vi "Thermostat.vi"() -> ()   [LabVIEW 2025]
panel:
  out "Week day":string
  out "Time":string
  out "Date":string
  out "Desired Temp":dbl format="%#_3g"
  out "Heater on":bool
  out "Room name":string
  out "Current Temp":dbl format="%#_3g"
  in  "STOP":bool
  in  "DOWN":bool
  in  "UP":bool
  in  "Room select":i32 min=0 max=3
  # "Set"
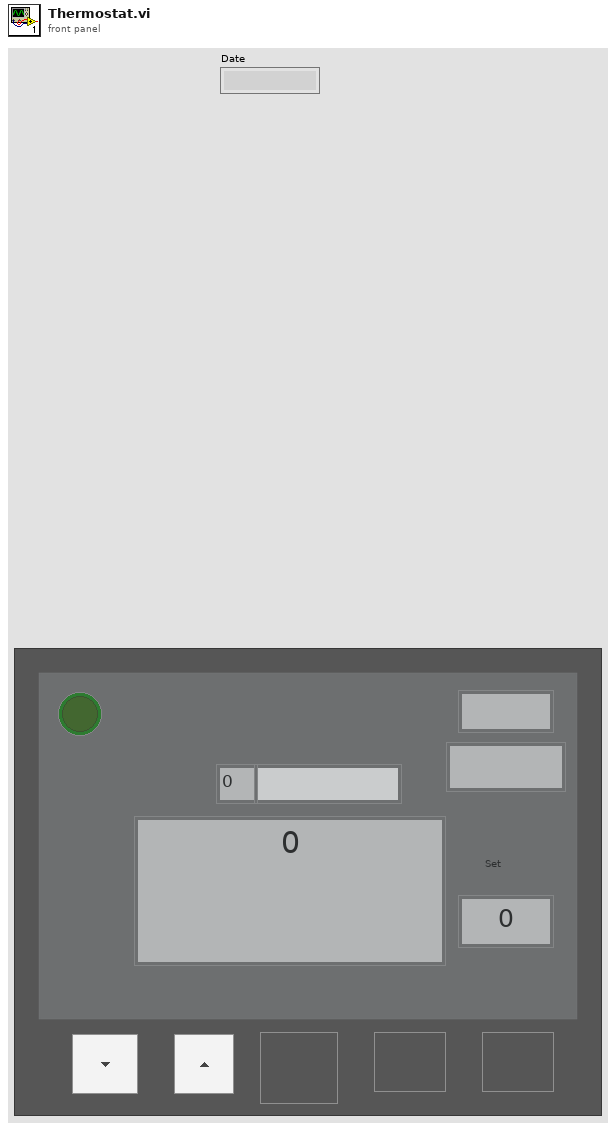
[diagram p1: front panel]
types:
  T1 = cluster{"Room name":string, "Desired Temp":dbl, "Current Temp":dbl, "Heater on":bool}[]
  T2 = cluster{"Room name":string, "Desired Temp":dbl, "Current Temp":dbl, "Heater on":bool}
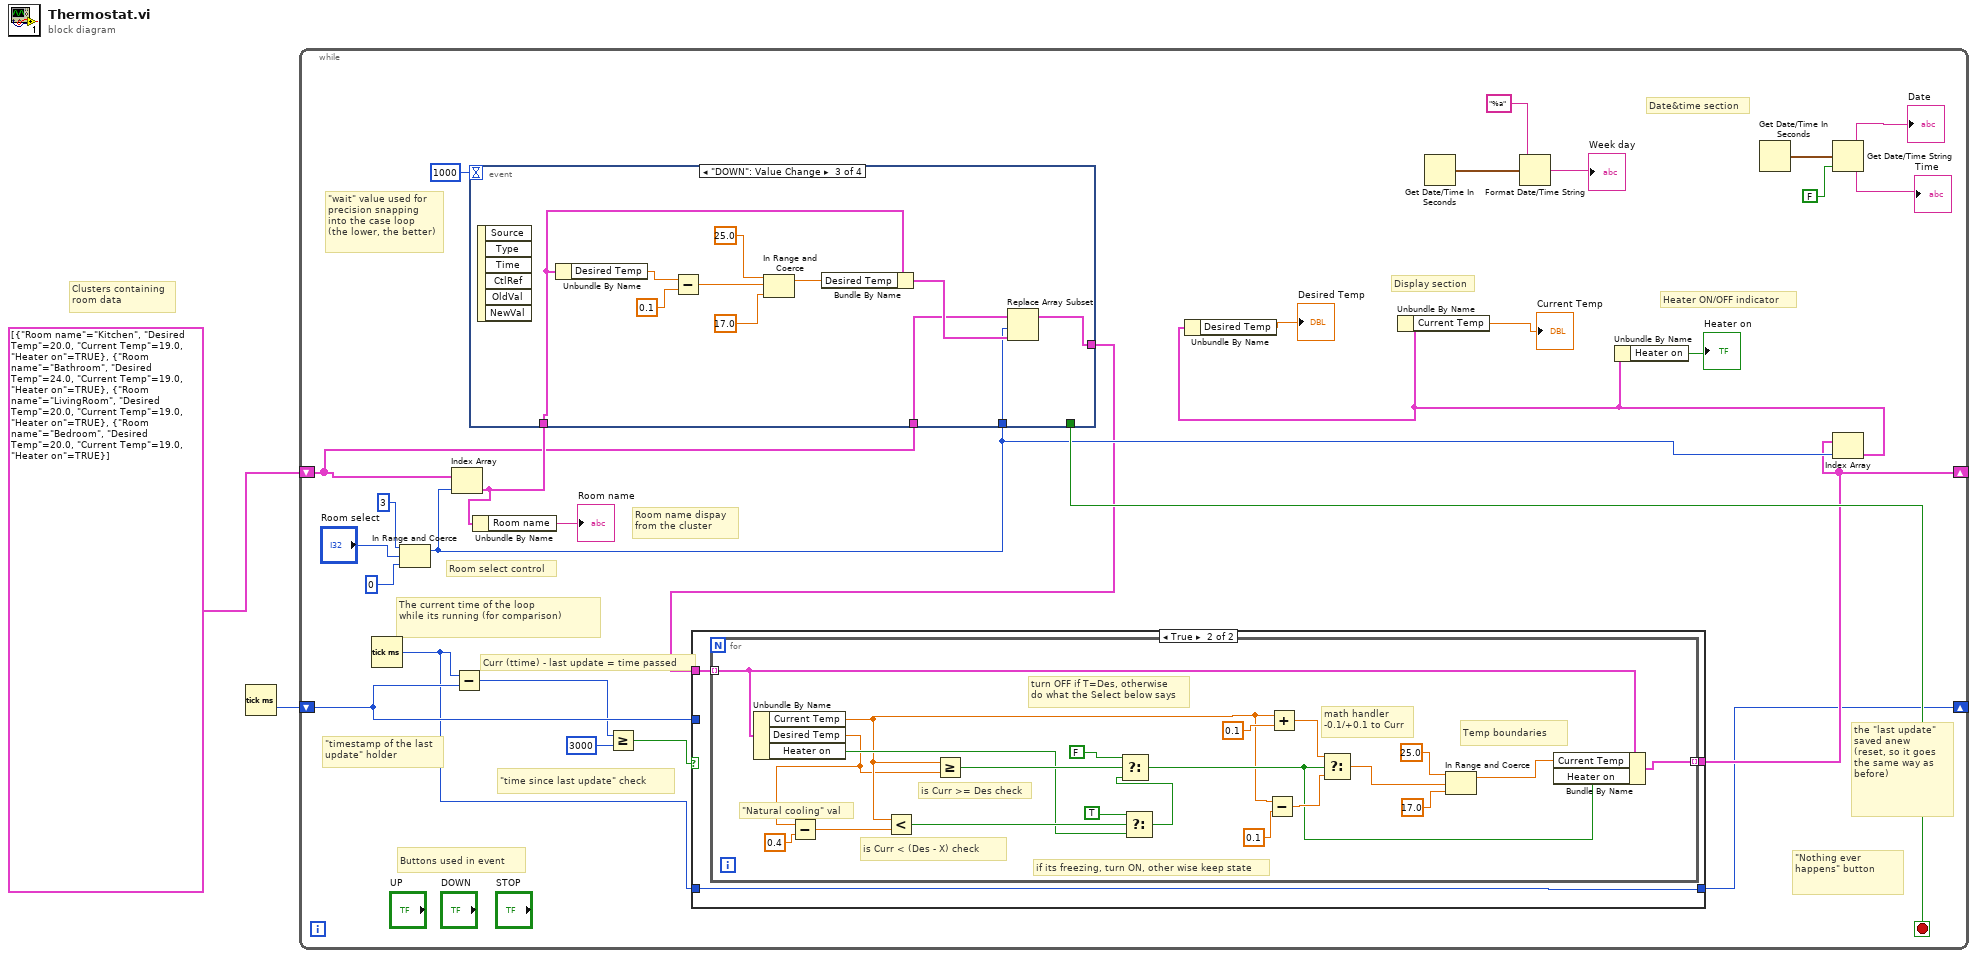
[diagram p0: block diagram]
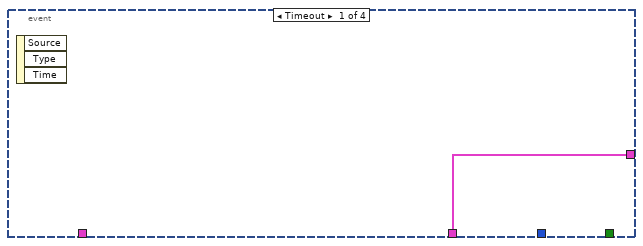
[diagram p3: hidden frame]
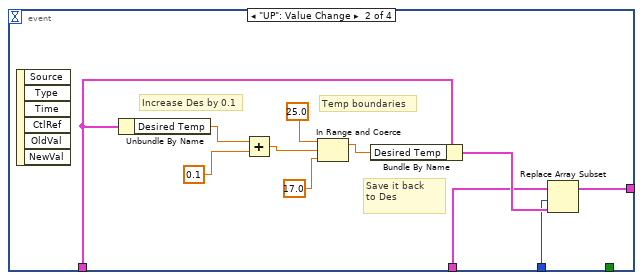
[diagram p4: hidden frame]
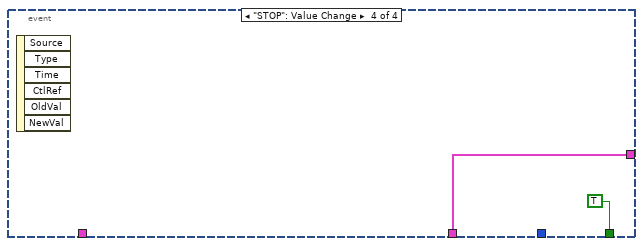
[diagram p5: hidden frame]
diagram:
  # "Clusters containing\nroom data"
  n1 = Tick Count (ms)() -> (millisecond timer value=w1:u32)
  n2 = while {
    shift-right: [w19] -> _
    shift-left: T1 [{"Room name"="Kitchen", "Desired Temp"=20.0, "Current Temp"=19.0, "Heater on"=TRUE}, {"Room name"="Bathroom", "Desired Temp"=24.0, "Current Temp"=19.0, "Heater on"=TRUE}, {"Room name"="LivingRoom", "Desired Temp"=20.0, "Current Temp"=19.0, "Heater on"=TRUE}, {"Room name"="Bedroom", "Desired Temp"=20.0, "Current Temp"=19.0, "Heater on"=TRUE}] -> [w20]
    shift-right: [w14] -> _
    shift-left: w1 -> [w16]
    stop <- w28 stop-if-true
    # "Heater ON/OFF indicator"
    # "Date&time section"
    # "Room select control"
    # "\"timestamp of the last\nupdate\" holder"
    # "\"wait\" value used for\nprecision snapping\ninto the case loop\n(the lower, the better)"
    # "the \"last update\"\nsaved anew\n(reset, so it goes\nthe same way as\nbefore)"
    # "\"time since last update\" check"
    # "Curr (ttime) - last update = time passed"
    # "The current time of the loop\nwhile its running (for comparison)"
    # "Buttons used in event"
    # "Room name dispay\nfrom the cluster"
    # "\"Nothing ever\nhappens\" button"
    # "Display section"
    n3 = Tick Count (ms)() -> (millisecond timer value=w13:u32)
    n4 = In Range and Coerce(upper limit=3, x="Room select", lower limit=0) -> (coerced(x)=w22:i32)  [unwired: 1 out]
    n5 = Index Array(array=w20, index=w22) -> (element=w23:T2)
    n6 = Subtract(x=w13, y=w16) -> (x-y=w15:u32)
    n7 = event shown="[2] \"DOWN\": Value Change" {
      selector: _ -> [_ _ _ _]
      dyn-events: _ -> [_ _ _ _]
      timeout: 1000 -> [_ _ _ _]
      tunnel: w23 -> [_ w63 w74 _]
      tunnel: [w57 w58 w70 w80] -> w12
      tunnel: w22 -> [_ w59 w69 _]
      tunnel: w20 -> [w57 w60 w71 w80]
      tunnel: [_ _ _ TRUE] -> w28
      event Timeout {
        n8 = event-data() -> ()  [unwired: 1 in, 3 out]
      }
      event "UP": Value Change {
        # "Save it back\nto Des"
        # "Increase Des by 0.1"
        # "Temp boundaries"
        n9 = event-data() -> ()  [unwired: 1 in, 6 out]
        n10 = Unbundle By Name(w63) -> ("Desired Temp"=w67:dbl)
        n11 = Add(x=w67, y=0.1) -> (x+y=w66:dbl)
        n12 = In Range and Coerce(upper limit=25.0, x=w66, lower limit=17.0) -> (coerced(x)=w62:dbl)  [unwired: 1 out]
        n13 = Bundle By Name(cluster=w63, "Desired Temp"=w62) -> (w61:T2)
        n14 = Replace Array Subset(array=w60, new element=w61, index=w59) -> (w58:T1)
      }
      event "DOWN": Value Change {
        n15 = event-data() -> ()  [unwired: 1 in, 6 out]
        n16 = Unbundle By Name(w74) -> ("Desired Temp"=w78:dbl)
        n17 = Subtract(x=w78, y=0.1) -> (x-y=w77:dbl)
        n18 = In Range and Coerce(upper limit=25.0, x=w77, lower limit=17.0) -> (coerced(x)=w73:dbl)  [unwired: 1 out]
        n19 = Bundle By Name(cluster=w74, "Desired Temp"=w73) -> (w72:T2)
        n20 = Replace Array Subset(array=w71, new element=w72, index=w69) -> (w70:T1)
      }
      event "STOP": Value Change {
        n21 = event-data() -> ()  [unwired: 1 in, 6 out]
      }
    }
    n22 = Unbundle By Name(w23) -> ("Room name"=→"Room name":string)
    n23 = Greater Or Equal?(x=w15, y=u32 3000) -> (x >= y?=w17:bool)
    n24 = case shown="True" w17 {
      tunnel: w12 -> [w32 w35]
      tunnel: [w32 w34] -> w19
      tunnel: w16 -> [w31 _]
      tunnel: w13 -> [_ w33]
      tunnel: [w31 w33] -> w14
      frame False {
      }
      frame True {
        n25 = for {
          tunnel: w35 -> [w39] mode=indexing
          tunnel: [w53] -> w34 mode=indexing
          # "Temp boundaries"
          # "math handler\n-0.1/+0.1 to Curr"
          # "turn OFF if T=Des, otherwise\ndo what the Select below says"
          # "if its freezing, turn ON, other wise keep state"
          # "\"Natural cooling\" val"
          # "is Curr < (Des - X) check"
          # "is Curr >= Des check"
          n26 = Unbundle By Name(w39) -> ("Current Temp"=w37:dbl, "Desired Temp"=w36:dbl, "Heater on"=w42:bool)
          n27 = Subtract(x=w36, y=0.4) -> (x-y=w51:dbl)
          n28 = Less?(x=w37, y=w51) -> (x < y?=w50:bool)
          n29 = Greater Or Equal?(x=w37, y=w36) -> (x >= y?=w48:bool)
          n30 = Select(t=TRUE, s=w50, f=w42) -> (s? t:f=w46:bool)
          n31 = Select(t=FALSE, s=w48, f=w46) -> (s? t:f=w38:bool)
          n32 = Subtract(x=w37, y=0.1) -> (x-y=w40:dbl)
          n33 = Add(x=w37, y=0.1) -> (x+y=w44:dbl)
          n34 = Select(t=w44, s=w38, f=w40) -> (s? t:f=w43:dbl)
          n35 = In Range and Coerce(upper limit=25.0, x=w43, lower limit=17.0) -> (coerced(x)=w56:dbl)  [unwired: 1 out]
          n36 = Bundle By Name(cluster=w39, "Current Temp"=w56, "Heater on"=w38) -> (w53:T2)
        }
      }
    }
    n37 = Get Date/Time In Seconds() -> (seconds since 1Jan1904=w10:timestamp)
    n38 = Format Date/Time String(time format string (%c)="%a", seconds (now)=w10) -> (date/time string=→"Week day":string)  [unwired: 1 in]
    n39 = Get Date/Time In Seconds() -> (seconds since 1Jan1904=w9:timestamp)
    n40 = Get Date/Time String(seconds (now)=w9, want seconds? (F)=FALSE) -> (date string=→"Date":string, time string=→"Time":string)  [unwired: 1 in]
    n41 = Index Array(array=w19, index=w22) -> (element=w4:T2)
    n42 = Unbundle By Name(w4) -> ("Desired Temp"=→"Desired Temp":dbl)
    n43 = Unbundle By Name(w4) -> ("Current Temp"=→"Current Temp":dbl)
    n44 = Unbundle By Name(w4) -> ("Heater on"=→"Heater on":bool)
  }
